vi "Add BrowerComponent.vi"(8 "error in (no error)":errorcluster, 9 "Parent Tag(\"\")":string, 10 "Builder":refnum<class "AbstractBuilder.lvclass">, 11 "BrowerController in":refnum<class "BrowerController.lvclass">) -> (0 "error out":errorcluster, 3 "BrowerController out":refnum<class "BrowerController.lvclass">)   [LabVIEW 2015, in "BrowerController.lvclass"]
uses:
  BrowerController.lvclass
  Models/BrowerBuilder/AbstractBuilder/AbstractBuilder.lvclass
  BrowerController.lvclass/BrowerController.ctl
  Models/BrowerTree/Type Definition/Symbol Index.ctl
  Models/BrowerComponent/BrowerComponent/BrowerComponent.lvclass
  Models/BrowerBuilder/BrowerGuidencer/BrowerGuidencer.lvclass
  Models/BrowerTree/BrowerTree.lvclass
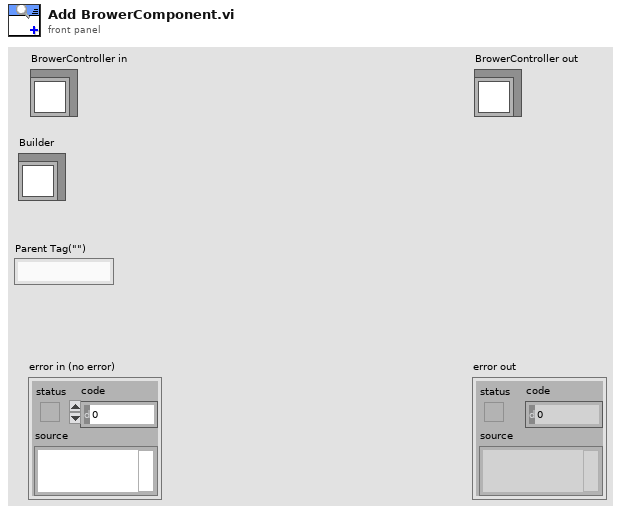
[diagram p1: front panel]
types:
  T1 = typedef "BrowerTree.lvclass/Symbol Index.ctl" = enum16{"PC", "Project", "Module", "DebugTask", "Communication"}
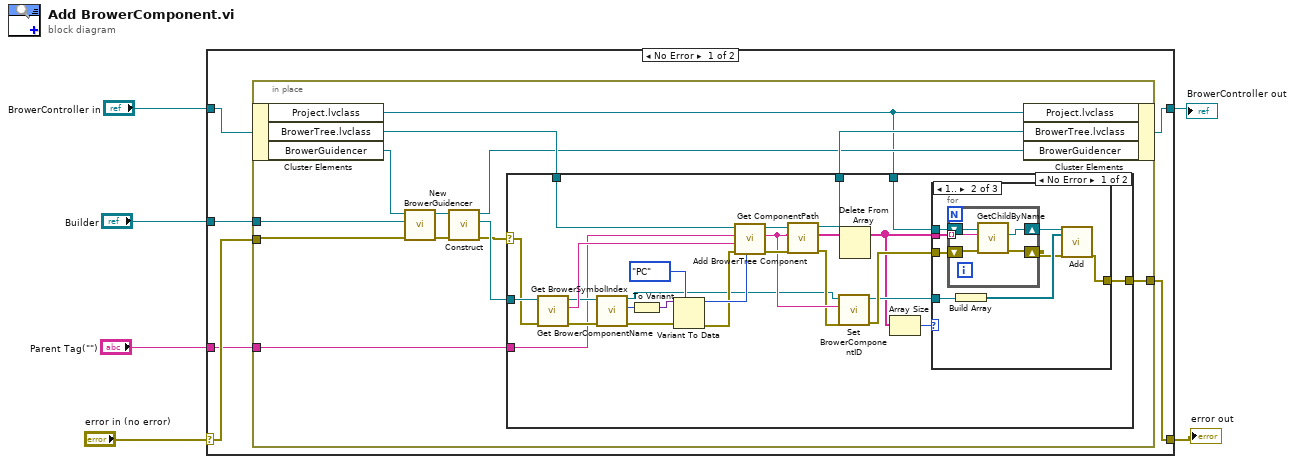
[diagram p0: block diagram]
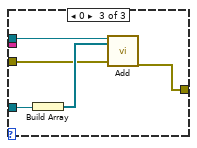
[diagram p3: hidden frame]
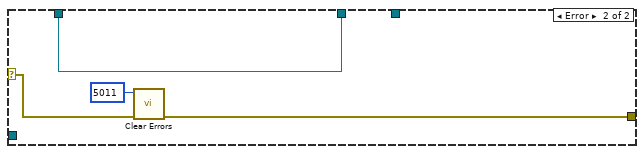
[diagram p4: hidden frame]
diagram:
  n1 = case shown="No Error" "error in (no error)" {
    selector: "error in (no error)" -> [w11 w76]
    tunnel: [w7 w76] -> w5
    tunnel: [w8 w75] -> w3
    tunnel: "BrowerController in" -> [w9 w75]
    tunnel: "Builder" -> [w12 _]
    tunnel: "Parent Tag(\"\")" -> [w10 _]
    frame No Error {
      n2 = in-place {
        in-place-border: w12 -> [w25]
        in-place-border: w11 -> [w24]
        in-place-border: w10 -> [w21]
        in-place-border: [w16] -> w7
        n3 = in-place-cluster #1(w9) -> ("Project.lvclass"=w13:refnum<class "BrowerComponent.lvclass">, "BrowerTree.lvclass"=w18:refnum<class "BrowerTree.lvclass">, "BrowerGuidencer"=w19:refnum<class "BrowerGuidencer.lvclass">)
        n4 = call "New BrowerGuidencer.vi"("error in (no error)"=w24, "AbstractBuilder"=w25, "reference in"=w19) -> ("error out"=w22:errorcluster, "reference out"=w23:refnum<class "BrowerGuidencer.lvclass">)  [unwired: 7 in]
        n5 = call "Construct.vi"("error in (no error)"=w22, "reference in"=w23) -> ("error out"=w14:errorcluster, "BrowerComponent"=w20:refnum<class "BrowerComponent.lvclass">, "reference out"=w15:refnum<class "BrowerGuidencer.lvclass">)  [unwired: 7 in]
        n6 = case shown="No Error" w14 {
          selector: w14 -> [w30 w73]
          tunnel: w21 -> [w29 _]
          tunnel: w20 -> [w51 _]
          tunnel: w18 -> [w49 w74]
          tunnel: [w42 w74] -> w17
          tunnel: [w41 w71] -> w16
          tunnel: w13 -> [w28 _]
          frame No Error {
            n7 = call "Get BrowerComponentName.vi"("error in (no error)"=w30, "BrowerComponent in"=w51) -> ("error out"=w38:errorcluster, "ComponentName"=w50:string, "BrowerComponent out"=w39:refnum<class "BrowerComponent.lvclass">)  [unwired: 7 in]
            n8 = call "Get BrowerSymbolIndex.vi"("error in (no error)"=w38, "BrowerComponent in"=w39) -> ("error out"=w36:errorcluster, "SymbolIndex"=w37:i32, "BrowerComponent out"=w31:refnum<class "BrowerComponent.lvclass">)  [unwired: 7 in]
            n9 = To Variant(anything=w37) -> (Variant=w35:variant)
            n10 = Variant To Data(error in=w36, type=Symbol_Index."PC" ("SymbolIndex"), Variant=w35) -> (data=w33:T1, error out=w32:errorcluster)
            n11 = call "Add BrowerTree Component.vi"("SymbolIndex"=w33, "error in (no error)"=w32, "Left Cell String"=w50, "Parent Tag"=w29, "BrowerTree in"=w49) -> ("error out"=w48:errorcluster, "BrowerComponentID(\"\")"=w46:string, "BrowerTree out"=w47:refnum<class "BrowerTree.lvclass">)  [unwired: 4 in]
            n12 = call "Get ComponentPath.vi"("error in (no error)"=w48, "BrowerComponentID(\"\")"=w46, "BrowerTree in"=w47) -> ("error out"=w45:errorcluster, "Navigate Tree:Get Paths"=w40:string[], "BrowerTree out"=w42:refnum<class "BrowerTree.lvclass">)  [unwired: 6 in]
            n13 = call "Set BrowerComponentID.vi"("error in (no error)"=w45, "ComponentID(\"\")"=w46, "BrowerComponent in"=w31) -> ("error out"=w44:errorcluster, "BrowerComponent out"=w43:refnum<class "BrowerComponent.lvclass">)  [unwired: 7 in]
            n14 = Delete From Array(array=w40) -> (array with subset deleted=w27:string[])  [unwired: 2 in, 1 out]
            n15 = Array Size(array=w27) -> (size(s)=w26:i32)
            n16 = case shown="1.." w26 {
              tunnel: w44 -> [w52 w60 w66]
              tunnel: w43 -> [_ w59 w70]
              tunnel: [w52 w58 w69] -> w41
              tunnel: w27 -> [_ w57 _]
              tunnel: w28 -> [_ w56 w67]
              frame Default {
              }
              frame 1.. {
                n17 = for {
                  tunnel: w57 -> [w64] mode=indexing
                  shift-right: [w61] -> w53
                  shift-left: w56 -> [w65]
                  shift-right: [w62] -> w54
                  shift-left: w60 -> [w63]
                  n18 = call-dynamic "GetChildByName.vi"("error in (no error)"=w63, "BrowerComponentID(\"\")"=w64, "reference in"=w65) -> ("error out"=w62:errorcluster, "BrowerComponent"=w61:refnum<class "BrowerComponent.lvclass">)  [unwired: 6 in, 1 out]
                }
                n19 = Build Array(w59) -> (w55:refnum<class "BrowerComponent.lvclass">[])
                n20 = call-dynamic "Add.vi"("reference in"=w53, "BrowerComponents"=w55, "error in (no error)"=w54) -> ("error out"=w58:errorcluster)  [unwired: 15 in, 1 out]
              }
              frame 0 {
                n21 = Build Array(w70) -> (w68:refnum<class "BrowerComponent.lvclass">[])
                n22 = call-dynamic "Add.vi"("reference in"=w67, "BrowerComponents"=w68, "error in (no error)"=w66) -> ("error out"=w69:errorcluster)  [unwired: 15 in, 1 out]
              }
            }
          }
          frame Error {
            n23 = call <vilib>:"Clear Errors.vi"("error in (no error)"=w73, "specific error code to clear (0: all)"=5011) -> ("error out"=w71:errorcluster)  [unwired: 4 in, 1 out]
          }
        }
        n24 = in-place-cluster #1("Project.lvclass"=w13, "BrowerTree.lvclass"=w17, "BrowerGuidencer"=w15) -> (w8:refnum<class "BrowerController.lvclass">)
      }
    }
    frame Error {
    }
  }
  "error out" <- w5
  "BrowerController out" <- w3
